vi "Untitled 1.vi"() -> ()   [LabVIEW 2021]
panel:
  in  "stop":bool
  out "A/DIO0 (Pin 11) 4":bool
  out "A/DIO0 (Pin 11) 3":bool
  out "A/DIO0 (Pin 11) 2":bool
  out "A/DIO0 (Pin 11)":bool
  in  "Double":dbl
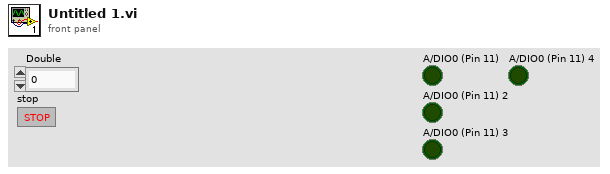
[diagram p1: front panel]
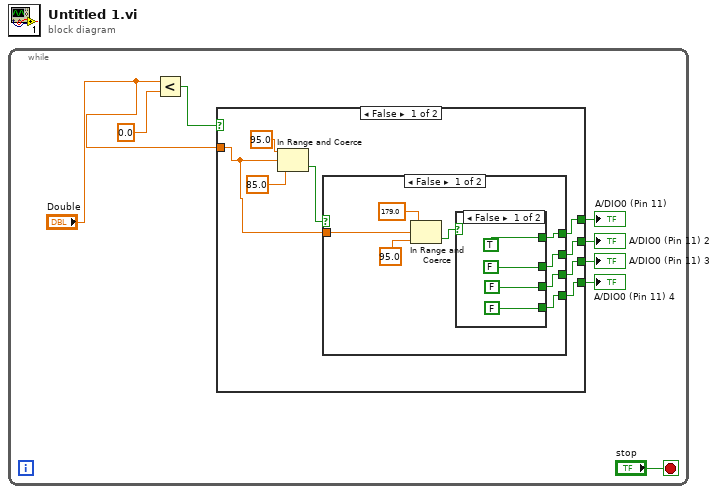
[diagram p0: block diagram]
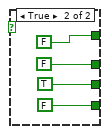
[diagram p2: hidden frame]
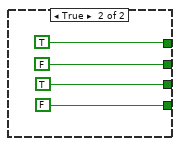
[diagram p3: hidden frame]
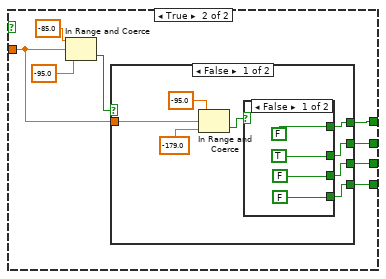
[diagram p4: hidden frame]
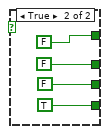
[diagram p5: hidden frame]
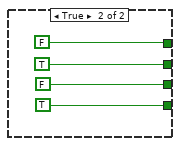
[diagram p6: hidden frame]
diagram:
  n1 = while {
    stop <- "stop" stop-if-true
    n2 = Less?(x="Double", y=0.0) -> (x < y?=w7:bool)
    n3 = case shown="False" w7 {
      tunnel: "Double" -> [w13 w41]
      tunnel: [w12 w38] -> w6
      tunnel: [w11 w40] -> w5
      tunnel: [w10 w39] -> w4
      tunnel: [w9 w37] -> w3
      frame False {
        n4 = In Range and Coerce(upper limit=95.0, x=w13, lower limit=85.0) -> (In Range?=w14:bool)  [unwired: 1 out]
        n5 = case shown="False" w14 {
          tunnel: w13 -> [w22 _]
          tunnel: [w20 FALSE ("A/DIO0 (Pin 11)")] -> w11
          tunnel: [w19 TRUE ("A/DIO0 (Pin 11)")] -> w10
          tunnel: [w18 TRUE ("A/DIO0 (Pin 11)")] -> w12
          tunnel: [w17 FALSE ("A/DIO0 (Pin 11)")] -> w9
          frame False {
            n6 = In Range and Coerce(upper limit=179.0, x=w22, lower limit=95.0) -> (In Range?=w21:bool)  [unwired: 1 out]
            n7 = case shown="False" w21 {
              tunnel: [TRUE ("A/DIO0 (Pin 11)") FALSE ("A/DIO0 (Pin 11)")] -> w18
              tunnel: [FALSE ("A/DIO0 (Pin 11)") FALSE ("A/DIO0 (Pin 11)")] -> w20
              tunnel: [FALSE ("A/DIO0 (Pin 11)") TRUE ("A/DIO0 (Pin 11)")] -> w19
              tunnel: [FALSE ("A/DIO0 (Pin 11)") FALSE ("A/DIO0 (Pin 11)")] -> w17
              frame False {
              }
              frame True {
              }
            }
          }
          frame True {
          }
        }
      }
      frame True {
        n8 = In Range and Coerce(upper limit=-85.0, x=w41, lower limit=-95.0) -> (In Range?=w42:bool)  [unwired: 1 out]
        n9 = case shown="False" w42 {
          tunnel: w41 -> [w50 _]
          tunnel: [w48 TRUE ("A/DIO0 (Pin 11)")] -> w40
          tunnel: [w47 FALSE ("A/DIO0 (Pin 11)")] -> w39
          tunnel: [w46 FALSE ("A/DIO0 (Pin 11)")] -> w38
          tunnel: [w45 TRUE ("A/DIO0 (Pin 11)")] -> w37
          frame False {
            n10 = In Range and Coerce(upper limit=-95.0, x=w50, lower limit=-179.0) -> (In Range?=w49:bool)  [unwired: 1 out]
            n11 = case shown="False" w49 {
              tunnel: [FALSE ("A/DIO0 (Pin 11)") FALSE ("A/DIO0 (Pin 11)")] -> w46
              tunnel: [TRUE ("A/DIO0 (Pin 11)") FALSE ("A/DIO0 (Pin 11)")] -> w48
              tunnel: [FALSE ("A/DIO0 (Pin 11)") FALSE ("A/DIO0 (Pin 11)")] -> w47
              tunnel: [FALSE ("A/DIO0 (Pin 11)") TRUE ("A/DIO0 (Pin 11)")] -> w45
              frame False {
              }
              frame True {
              }
            }
          }
          frame True {
          }
        }
      }
    }
    "A/DIO0 (Pin 11)" <- w6
    "A/DIO0 (Pin 11) 2" <- w5
    "A/DIO0 (Pin 11) 3" <- w4
    "A/DIO0 (Pin 11) 4" <- w3
  }
